vi "Send.vi"(7 "Device Address":u8, 8 "error in (no error)":errorcluster, 9 "eI2Cflags":T1 caption="I2C Flags" items=["None"=0, "START"=2, "REPEATED START"=3, "STOP"=4, "START AND STOP"=6], 10 "Buffer":u8[](array[numeric]), 11 "I2COUSBSim in":refnum<class "I2COUSBSim.lvclass">) -> (0 "error out":errorcluster, 1 "Status":string, 2 "Byte Returned":u32, 3 "I2COUSBSim out":refnum<class "I2COUSBSim.lvclass">)   [LabVIEW 2020, in "I2COUSB.lvlib" / "I2COUSBSim.lvclass"]
doc: "Send Data"
uses:
  I2COUSBSim.lvclass
  II2COUSB/TypeDef/I2CFlags.ctl
  I2COUSBSim.lvclass/I2COUSBSim.ctl
  II2COUSB/TypeDef/II2COUSB_typedef.lvlib
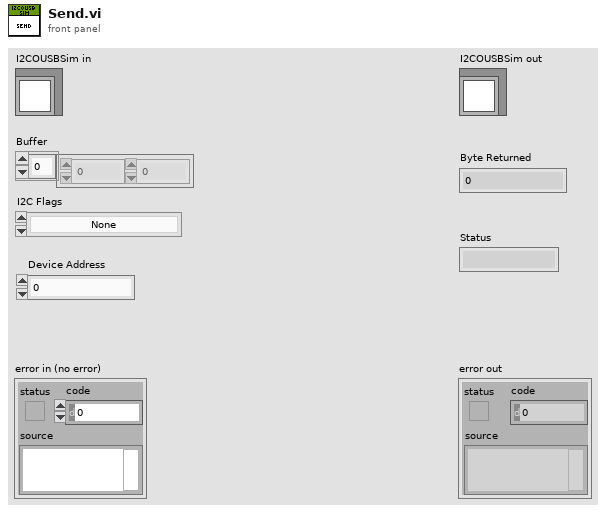
[diagram p1: front panel]
types:
  T1 = typedef "II2COUSB_typedef.lvlib/I2CFlags.ctl" = u8
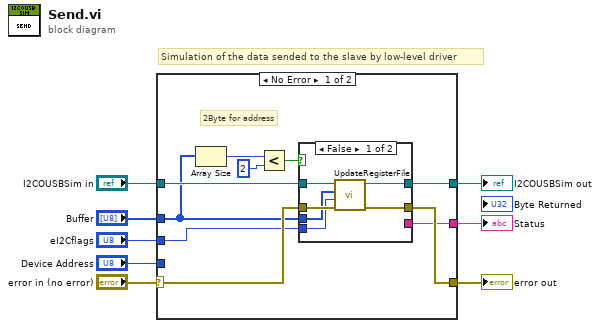
[diagram p0: block diagram]
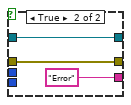
[diagram p2: hidden frame]
diagram:
  # "Simulation of the data sended to the slave by low-level driver"
  n1 = case shown="No Error" "error in (no error)" {
    selector: "error in (no error)" -> [w15 w28]
    tunnel: "I2COUSBSim in" -> [w13 w29]
    tunnel: [w12 w29] -> w7
    tunnel: [w14 w28] -> w5
    tunnel: "Buffer" -> [w10 _]
    tunnel: "eI2Cflags" -> [w11 _]
    tunnel: "Device Address" -> [_ _]
    tunnel: [w9 _] -> w1
    frame No Error {
      # "2Byte for address"
      n2 = Array Size(array=w10) -> (size(s)=w18:i32)
      n3 = Less?(x=w18, y=2) -> (x < y?=w16:bool)
      n4 = case shown="False" w16 {
        tunnel: w15 -> [w24 w27]
        tunnel: [w23 w27] -> w14
        tunnel: w13 -> [w22 w26]
        tunnel: [w21 w26] -> w12
        tunnel: w11 -> [w20 _]
        tunnel: w10 -> [w19 _]
        tunnel: [_ "Error"] -> w9
        frame False {
          n5 = call "UpdateRegisterFile.vi"("error in (no error)"=w24, "eI2Cflags"=w20, "Buffer"=w19, "I2COUSBSim in"=w22) -> ("error out"=w23:errorcluster, "I2COUSBSim out"=w21:refnum<class "I2COUSBSim.lvclass">)  [unwired: 6 in]
        }
        frame True {
        }
      }
    }
    frame Error {
    }
  }
  "error out" <- w5
  "I2COUSBSim out" <- w7
  "Status" <- w1
